vi "Calc - PSAVG.vi"(11 "00-01-9220":dbl[](array[numeric])) -> (3 "PSAvg":dbl format="%0.2f")   [LabVIEW 2018, in "Controller (Host).lvlib"]
uses:
  Controller (Host).lvlib
  <vilib>/Analysis/baseanly.llb/Mean (DBL).vi
  <vilib>/Analysis/NI_AALBase.lvlib
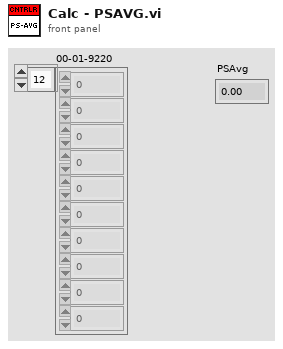
[diagram p1: front panel]
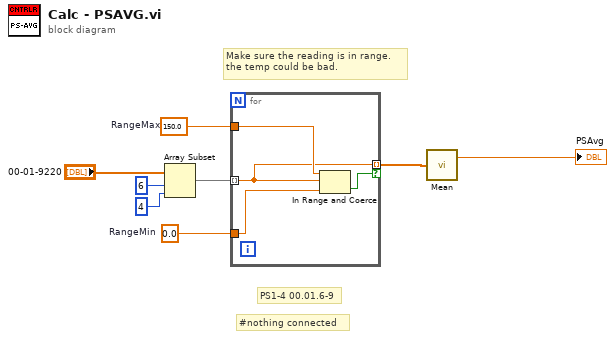
[diagram p0: block diagram]
diagram:
  w3 = 150.0  # RangeMax
  w4 = 0.0  # RangeMin
  # "#nothing connected"
  # "PS1-4 00.01.6-9"
  # "Make sure the reading is in range. \nthe temp could be bad."
  n1 = Array Subset(array="00-01-9220", index=6, length=4) -> (w5:dbl[])
  n2 = for {
    tunnel: w5 -> [w10] mode=indexing
    tunnel: w4 -> [w11]
    tunnel: w3 -> [w12]
    tunnel: [w10] -> w2 mode=indexing if=w9
    n3 = In Range and Coerce(upper limit=w12, x=w10, lower limit=w11) -> (In Range?=w9:bool)  [unwired: 1 out]
  }
  n4 = call-poly <vilib>:"Mean.vi"("X"=w2) -> ("mean"=→"PSAvg":dbl)  [unwired: 1 out]
